vi "Mock Call.vi"(8 "error in (no error)":errorcluster, 10 "VI Called":refnum<vi>, 11 "Mock In":refnum<class "Responsive Mock.lvclass">) -> (0 "error out":errorcluster, 3 "Mock Out":refnum<class "Responsive Mock.lvclass">)   [LabVIEW 2020, in "Responsive Mock.lvclass"]
uses:
  Responsive Mock.lvclass
  Responsive Mock.lvclass/Responsive Mock.ctl
  VI Server VI Call/VI Server VI Call.lvclass
  C:/git/astemes-lmock/source/Core/VI Call/VI Call.lvclass
  VI Server VI Call/Create.vi
  Core/Expectation/Expectation.lvclass
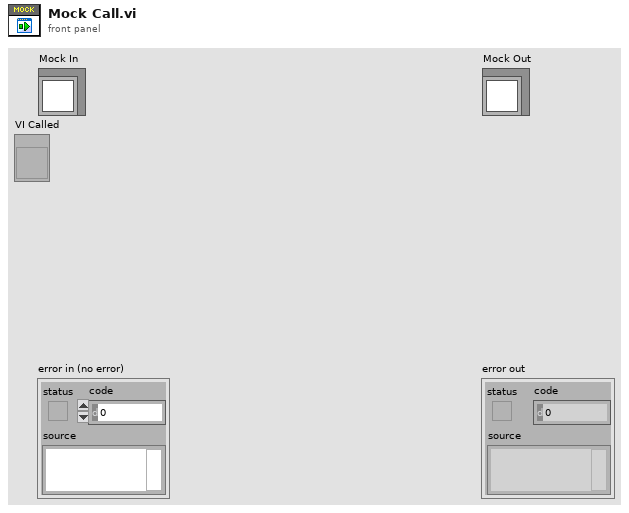
[diagram p1: front panel]
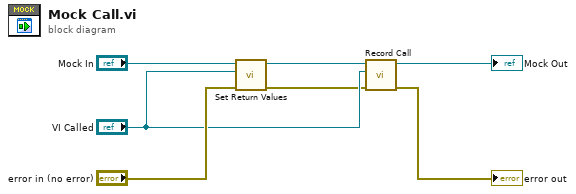
[diagram p0: block diagram]
diagram:
  n1 = call "Set Return Values.vi"("error in (no error)"="error in (no error)", "VI Reference"="VI Called", "Mock In"="Mock In") -> ("error out"=w2:errorcluster, "Mock Out"=w1:refnum<class "Responsive Mock.lvclass">)  [unwired: 7 in]
  n2 = call "Record Call.vi"("error in (no error)"=w2, "This VI"="VI Called", "Mock In"=w1) -> ("error out"=→"error out":errorcluster, "Mock Out"=→"Mock Out":refnum<class "Responsive Mock.lvclass">)  [unwired: 7 in]
